vi "DHE_Getfd.vi"(10 "DHE_Devices":T1[](array[typedef]) {"readtime" format="%.2f"}, 11 "cmd in":string) -> (1 "devname":string, 2 "fd":i32, 3 "cmd out":string, 4 "fpa":string, 5 "devno":i32, 6 "found":bool, 7 "index":i32)   [LabVIEW 2016]
uses:
  DHE_Device.ctl
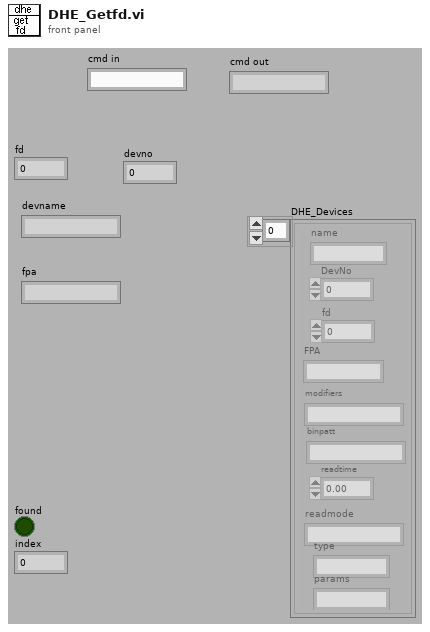
[diagram p1: front panel]
types:
  T1 = typedef "DHE_Device.ctl" = cluster{"DevNo":i32, "fd":i32, "name":string, "FPA":string, "modifiers":string, "binpatt":string, "readtime":dbl, "readmode":string, "type":string, "params":string}
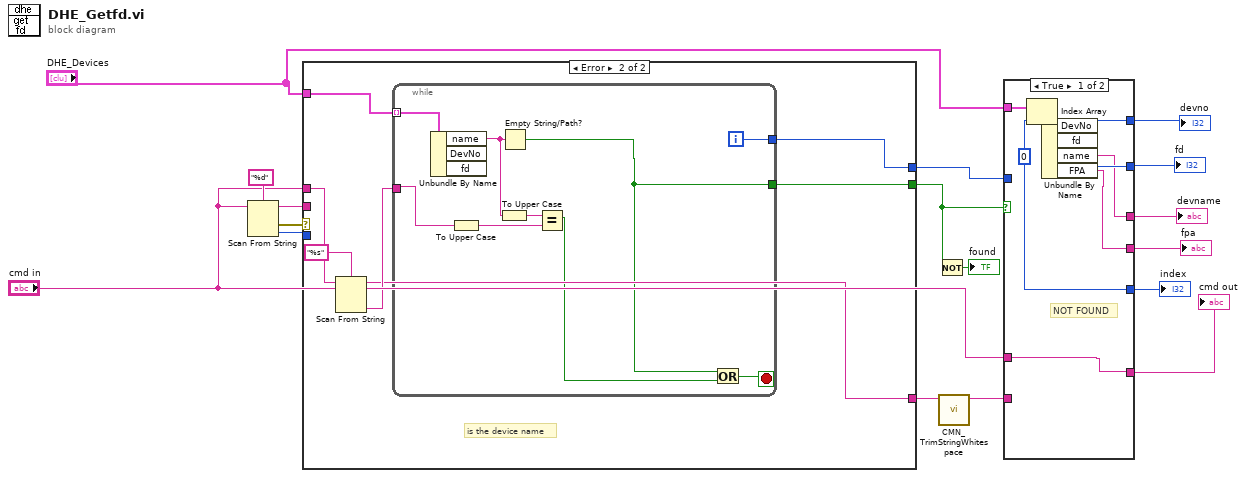
[diagram p0: block diagram]
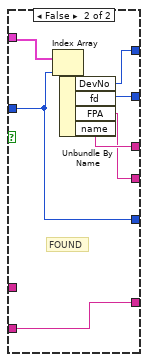
[diagram p2: hidden frame]
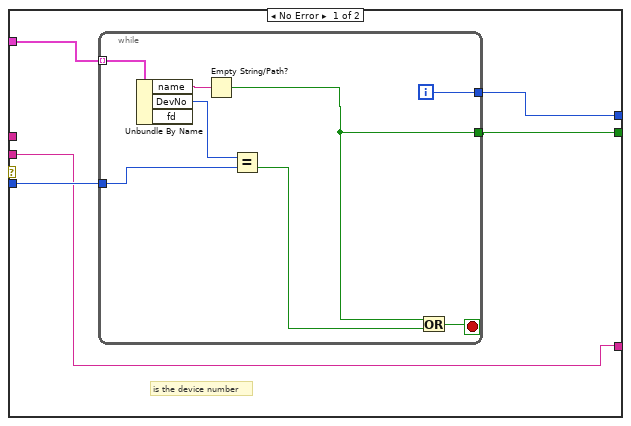
[diagram p3: hidden frame]
diagram:
  n1 = Scan From String(format string="%d", input string="cmd in") -> (remaining string=w10:string, error out=w14:errorcluster, output 1=w13:i32)  [unwired: 2 in, 2 out]
  n2 = case shown="Error" w14 {
    tunnel: "DHE_Devices" -> [w21 w37]
    tunnel: w13 -> [w22 _]
    tunnel: "cmd in" -> [_ w35]
    tunnel: [w20 w36] -> w8
    tunnel: [w18 w31] -> w2
    tunnel: [w19 w32] -> w12
    tunnel: w10 -> [w19 _]
    frame No Error {
      # "is the device number"
      n3 = while {
        tunnel: w21 -> [w30] mode=indexing
        tunnel: w22 -> [w28]
        tunnel: [w24] -> w20
        tunnel: [w23] -> w18
        i -> [w23]
        stop <- w25 stop-if-true
        n4 = Unbundle By Name(w30) -> ("name"=w27:string, "DevNo"=w29:i32)  [unwired: 1 out]
        n5 = Empty String/Path?(string/path=w27) -> (empty?=w24:bool)
        n6 = Equal?(x=w29, y=w28) -> (x = y?=w26:bool)
        n7 = Or(x=w24, y=w26) -> (x .or. y?=w25:bool)
      }
    }
    frame Error {
      # "is the device name"
      n8 = Scan From String(format string="%s", input string=w35) -> (remaining string=w32:string, output 1=w33:string)  [unwired: 2 in, 3 out]
      n9 = while {
        tunnel: w37 -> [w46] mode=indexing
        tunnel: [w43] -> w36
        tunnel: w33 -> [w41]
        tunnel: [w40] -> w31
        i -> [w40]
        stop <- w44 stop-if-true
        n10 = Unbundle By Name(w46) -> ("name"=w42:string)  [unwired: 2 out]
        n11 = To Upper Case(1:w41) -> (0:w38:string)
        n12 = To Upper Case(1:w42) -> (0:w39:string)
        n13 = Empty String/Path?(string/path=w42) -> (empty?=w43:bool)
        n14 = Equal?(x=w39, y=w38) -> (x = y?=w45:bool)
        n15 = Or(x=w43, y=w45) -> (x .or. y?=w44:bool)
      }
    }
  }
  n16 = Not(x=w8) -> (.not. x?=→"found":bool)
  n17 = call "CMN_TrimStringWhitespace.vi"("string"=w12) -> ("trimmed string"=w11:string)  [unwired: 1 in, 8 out]
  n18 = case shown="True" w8 {
    tunnel: [w54 w59] -> w17
    tunnel: [w50 w62] -> w16
    tunnel: w2 -> [_ w55]
    tunnel: w11 -> [_ w62]
    tunnel: "cmd in" -> [w50 _]
    tunnel: "DHE_Devices" -> [w53 w61]
    tunnel: [w49 w58] -> w7
    tunnel: [w48 w57] -> w6
    tunnel: [w47 w56] -> w5
    tunnel: [w52 w55] -> w1
    frame True {
      w52 = 0 ("index")
      # "NOT FOUND"
      n19 = Index Array(array=w53, index=w52) -> (element=w51:T1)
      n20 = Unbundle By Name(w51) -> ("DevNo"=w47:i32, "fd"=w54:i32, "name"=w49:string, "FPA"=w48:string)
    }
    frame False {
      # "FOUND"
      n21 = Index Array(array=w61, index=w55) -> (element=w60:T1)
      n22 = Unbundle By Name(w60) -> ("DevNo"=w56:i32, "fd"=w59:i32, "FPA"=w57:string, "name"=w58:string)
    }
  }
  "fd" <- w17
  "cmd out" <- w16
  "devname" <- w7
  "fpa" <- w6
  "devno" <- w5
  "index" <- w1
